vi "Main.vi"() -> ()   [LabVIEW 2010]
uses:
  typedefs/state_cluster.ctl
  typedefs/state_enum.ctl
  <vilib>/DAQmx/write.llb/DAQmx Write (Analog 1D DBL NChan 1Samp).vi
  <vilib>/DAQmx/create/channels.llb/DAQmx Create Channel (AO-Voltage-Basic).vi
  <vilib>/DAQmx/configure/timing.llb/DAQmx Timing (Sample Clock).vi
  <vilib>/DAQmx/miscellaneous.llb/DAQmx Fill In Error Info.vi
panel:
  in  "Zeit pro Zelle":dbl
  out "Internal quit":bool
  out "Pfadlänge":dbl
  out "Image":picture
  in  "Quit":bool
  out "Signal Qualität":dbl(slide) scale=0.0..10.0
  out "Anzahl Neurone":u16(slide) scale=0.0..200.0
  out "Scan Geschwindigkeit":dbl(slide) scale=0.0..1.0
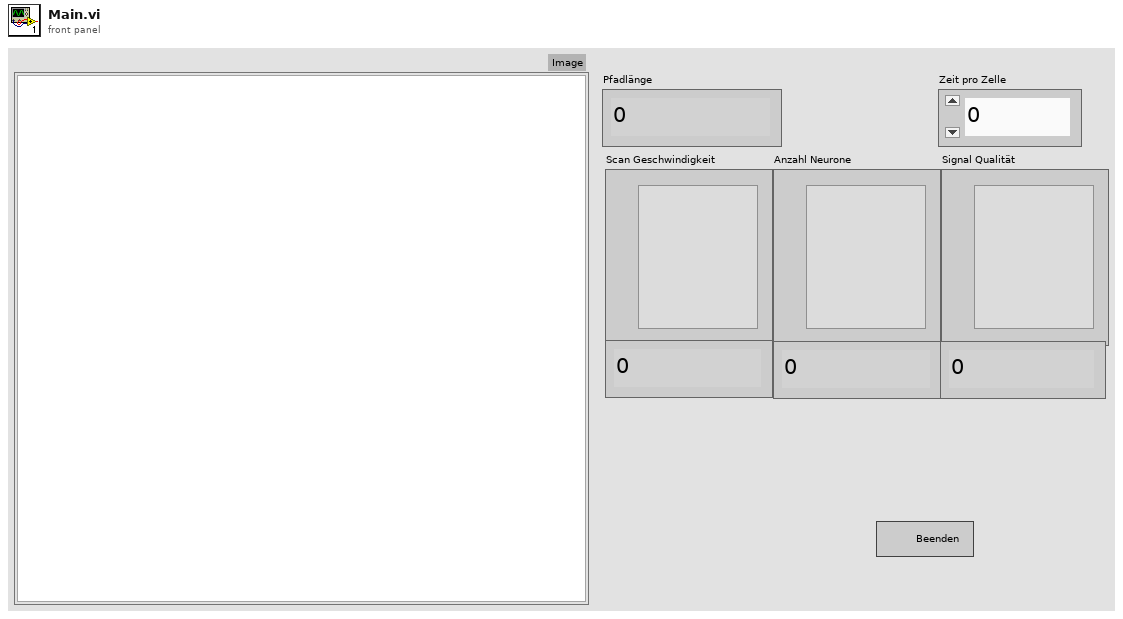
[diagram p1: front panel]
types:
  T1 = typedef "state_cluster.ctl" = cluster{"State":T2, "variant":variant}
  T2 = typedef "state_enum.ctl" = enum16{"Init", "StartSetting", "Moving", "SetNeuron", "FinishSetting", "Quit"}
  T3 = cluster{"Width":u16, "Style":enum32{"Solid", "Dash", "Dot", "DashDot", "DashDotDot"}}
  T4 = typedef "LVBoundsTypeDef.ctl" = cluster{"Width":u32, "Height":u32}
  T5 = typedef "LVMouseTypeDef.ctl" = cluster{"Mouse Position":cluster{"X":i32, "Y":i32}, "Mouse Modifiers":cluster{"Button Down":bool, "Shift Mod":bool, "Menu Mod":bool, "Option Mod":bool}}
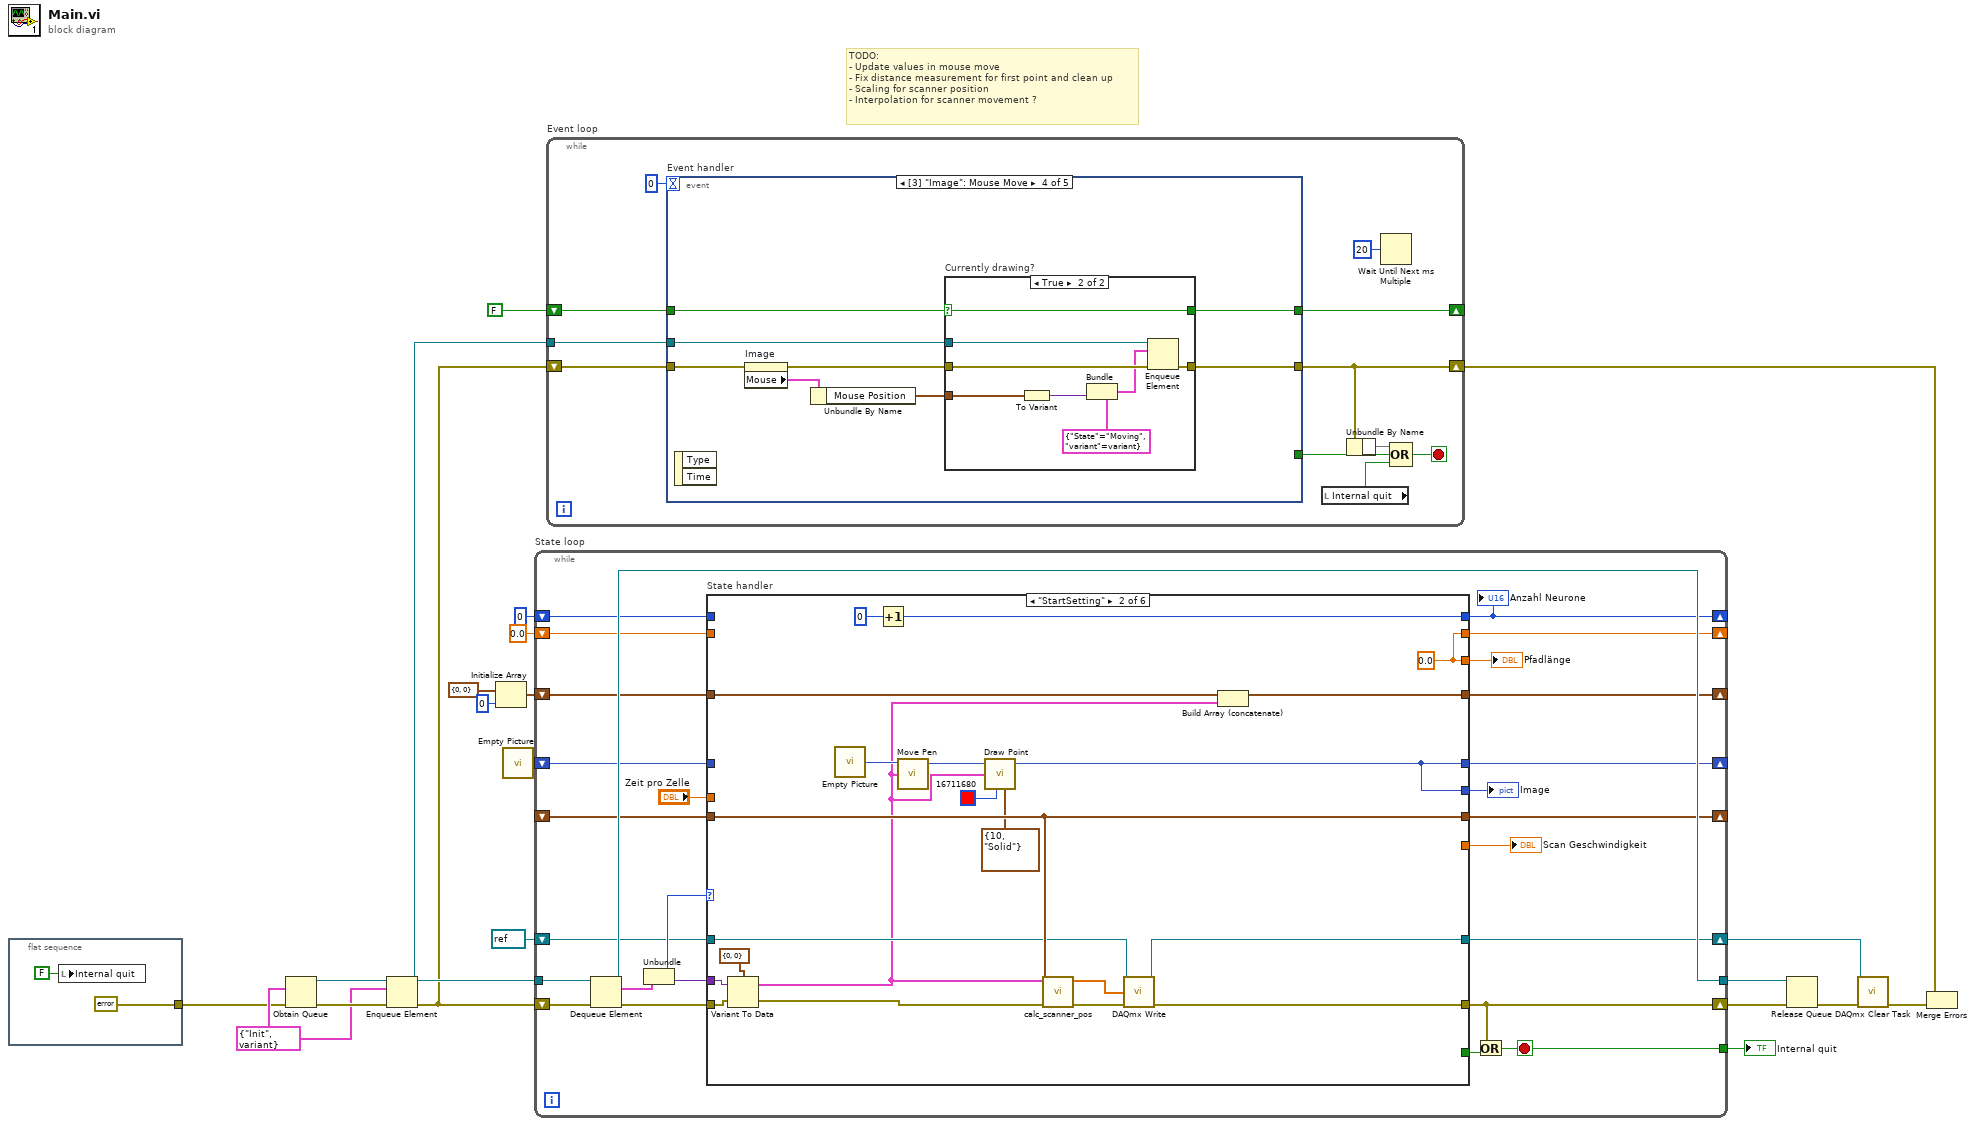
[diagram p0: block diagram]
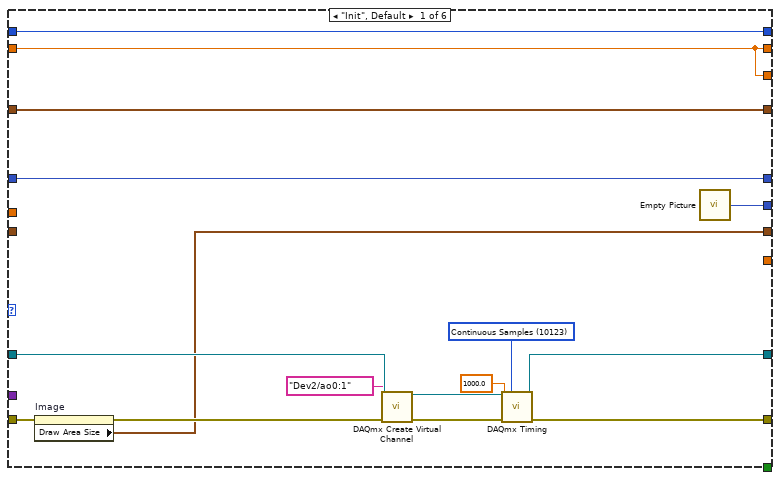
[diagram p2: hidden frame]
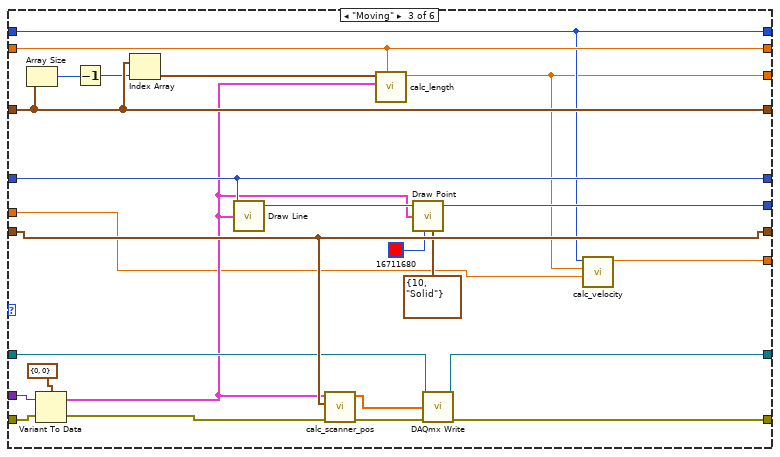
[diagram p3: hidden frame]
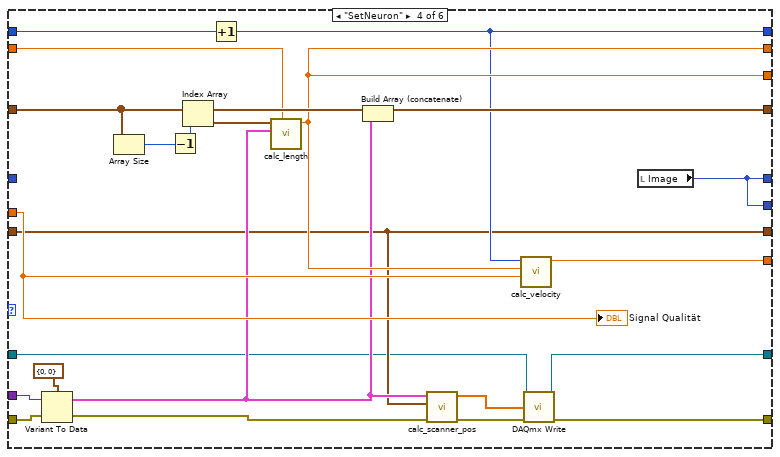
[diagram p4: hidden frame]
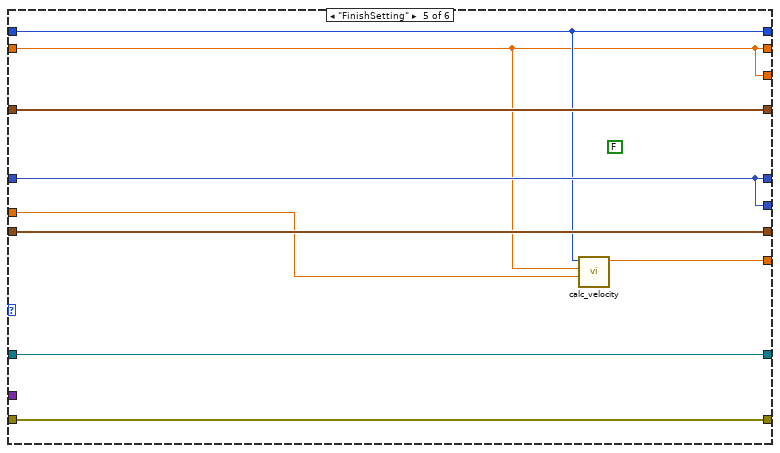
[diagram p5: hidden frame]
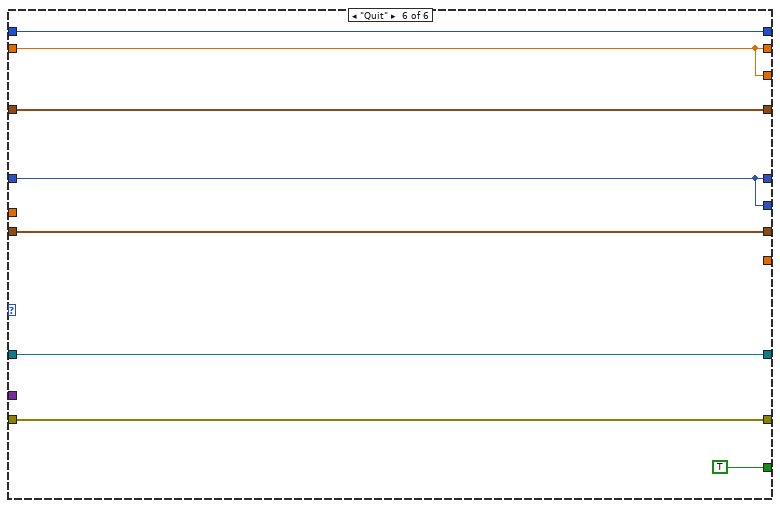
[diagram p6: hidden frame]
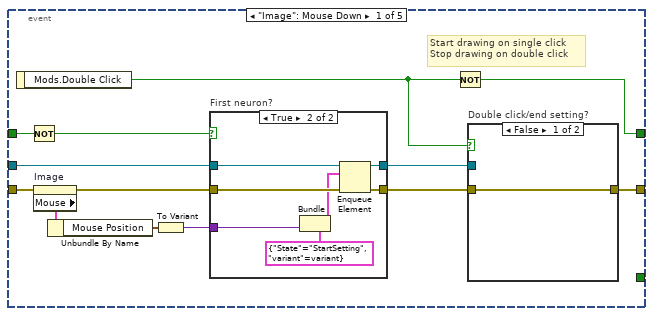
[diagram p7: hidden frame]
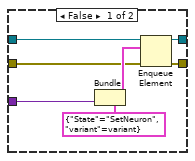
[diagram p8: hidden frame]
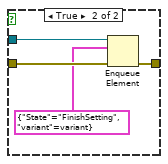
[diagram p9: hidden frame]
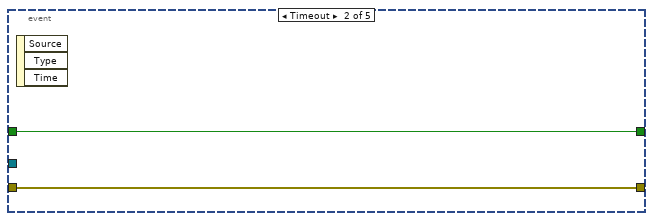
[diagram p10: hidden frame]
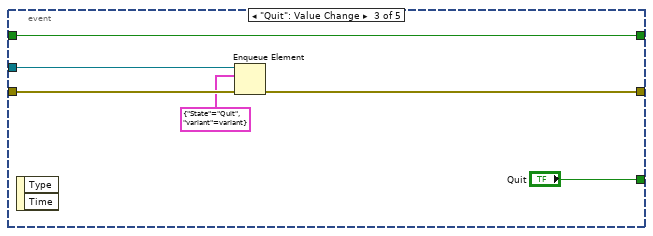
[diagram p11: hidden frame]
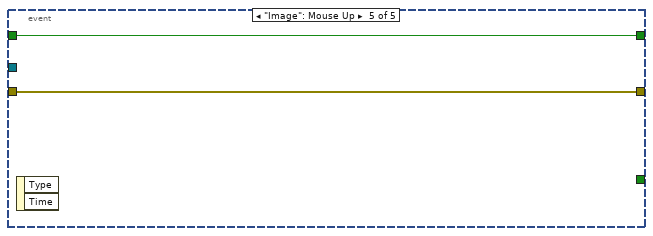
[diagram p13: hidden frame]
diagram:
  w18 = T1 {"State"=enum."Init", "variant"=variant}
  # "TODO:\n- Update values in mouse move\n- Fix distance measurement for first point and clean up\n- Scaling for scanner position\n- Interpolation for scanner movement ?"
  n1 = flat-sequence {
    tunnel: [errorcluster {"status"=FALSE, "code"=0, "source"=""} ("error in (no error)")] -> w5
    frame #0 {
      n2 = local write "Internal quit"(FALSE ("Internal quit")) -> ()
    }
  }
  n3 = Obtain Queue(element data type=w18, error in (no error)=w5) -> (queue out=w19:refnum<queue>, error out=w20:errorcluster)  [unwired: 3 in, 1 out]
  n4 = Enqueue Element(queue=w19, element=w18, error in (no error)=w20) -> (queue out=w10:refnum<queue>, error out=w8:errorcluster)  [unwired: 1 in, 1 out]
  n5 = Initialize Array(cluster{"X":i32, "Y":i32} {"X"=0, "Y"=0} ("Mouse Position"), 0 ("dimension size")) -> (w11:cluster{"X":i32, "Y":i32}[])
  n6 = call "Empty Picture"() -> ("empty picture"=w9:picture)
  n7 = while "State loop" {
    shift-right: [w42] -> w17
    shift-left: w8 -> [w49]
    tunnel: w10 -> [w47]
    tunnel: [w43] -> w16
    shift-right: [w30] -> _
    shift-left: u16 0 -> [w40]
    shift-right: [w34] -> _
    shift-left: 0.0 -> [w39]
    shift-right: [w37] -> _
    shift-left: w11 -> [w38]
    shift-right: [w35] -> _
    shift-left: w9 -> [w36]
    tunnel: [w31] -> w7
    shift-right: [w28] -> w1
    shift-left: refnum<k21> refnum ("task out") -> [w27]
    shift-right: [w26] -> _
    shift-left: _ -> [w25]
    stop <- w31 stop-if-true
    n8 = Dequeue Element(queue=w47, error in (no error)=w49) -> (queue out=w43:refnum<queue>, element=w46:T1, error out=w48:errorcluster)  [unwired: 1 in, 1 out]
    n9 = Unbundle(w46) -> ("State"=w45:T2, "variant"=w44:variant)
    n10 = case "State handler" shown="\"StartSetting\"" w45 {
      tunnel: w48 -> [w57 w85 w110 w133 w143 w145]
      tunnel: [w60 w77 w100 w118 w143 w145] -> w42
      tunnel: w44 -> [_ w84 w109 w132 _ _]
      tunnel: [_ _ _ _ _ TRUE] -> w41
      tunnel: w40 -> [w65 _ w89 w134 w137 w150]
      tunnel: [w65 w81 w89 w122 w137 w150] -> w30
      tunnel: w39 -> [w62 _ w107 w128 w136 w148]
      tunnel: w38 -> [w64 w72 w106 w129 w142 w149]
      tunnel: [w64 w73 w106 w130 w142 w149] -> w37
      tunnel: [w62 w82 w107 w123 w136 w148] -> w34
      tunnel: w36 -> [w63 _ w108 _ w141 w147]
      tunnel: [w63 w70 w108 w127 w141 w147] -> w35
      tunnel: [w61 w70 w94 w127 w141 w147] -> w33
      tunnel: [w62 w82 w88 w123 w136 w148] -> w32
      tunnel: "Zeit pro Zelle" -> [_ _ w87 w121 w135 _]
      tunnel: [w59 w75 w97 w114 w140 w146] -> w28
      tunnel: w27 -> [w58 w76 w98 w115 w140 w146]
      tunnel: [w55 w79 w99 w116 w139 w144] -> w26
      tunnel: w25 -> [_ w79 w99 w116 w139 w144]
      tunnel: [_ _ w90 w112 w138 _] -> w24
      frame "Init", Default {
        w53 = 10123 items=["Finite Samples"=10178, "Continuous Samples"=10123, "Hardware Timed Single Point"=12522] ("sample mode")
        n11 = property on="Image" class="Pict"(error in=w57) -> (error out=w56:errorcluster, "Draw Area Size"=w55:T4)  [unwired: 1 in, 1 out]
        n12 = call-poly <vilib>:"DAQmx Create Virtual Channel.vi"("task in"=w58, "physical channels"=tag "Dev2/ao0:1", "error in"=w56) -> ("task out"=w52:refnum<k21>, "error out"=w54:errorcluster)  [unwired: 11 in]
        n13 = call-poly <vilib>:"DAQmx Timing.vi"("task/channels in"=w52, "sample mode"=w53, "rate"=1000.0, "error in"=w54) -> ("task out"=w59:refnum<k21>, "error out"=w60:errorcluster)  [unwired: 10 in]
        n14 = call "Empty Picture"() -> ("empty picture"=w61:picture)
      }
      frame "StartSetting" {
        w82 = 0.0
        n15 = Variant To Data(error in=w85, Variant=w84, type=cluster{"X":i32, "Y":i32} {"X"=0, "Y"=0} ("Mouse Position")) -> (error out=w80:errorcluster, data=w69:cluster{})
        n16 = call "Empty Picture"() -> ("empty picture"=w83:picture)
        n17 = Increment(x=u16 0) -> (x+1=w81:u16)
        n18 = call <vilib>:"Move Pen.vi"("new position"=w69, "picture"=w83) -> ("new picture"=w71:picture)  [unwired: 3 in]
        n19 = call <vilib>:"Draw Point.vi"("picture"=w71, "point(x,y)"=w69, "color(black)"=u32 16711680, "pen"=T3 {"Width"=10, "Style"=enum."Solid"}) -> ("new picture"=w70:picture)  [unwired: 5 in]
        n20 = call "calc_scanner_pos.vi"("error in (no error)"=w80, "Draw Area Size"=w79, "Mouse position"=w69) -> ("error out"=w78:errorcluster, "Scanner position"=w74:dbl[])  [unwired: 7 in]
        n21 = call-poly <vilib>:"DAQmx Write.vi"("task/channels in"=w76, "data"=w74, "error in"=w78) -> ("task out"=w75:refnum<k21>, "error out"=w77:errorcluster)  [unwired: 10 in, 1 out]
        n22 = Build Array (concatenate)(w72, w69) -> (w73:cluster{"X":i32, "Y":i32}[])
      }
      frame "Moving" {
        n23 = Array Size(array=w106) -> (size(s)=w105:i32)
        n24 = Variant To Data(error in=w110, Variant=w109, type=cluster{"X":i32, "Y":i32} {"X"=0, "Y"=0} ("Mouse Position")) -> (error out=w101:errorcluster, data=w93:cluster{})
        n25 = Decrement(x=w105) -> (x-1=w104:i32)
        n26 = Index Array(array=w106, index=w104) -> (element=w103:cluster{"X":i32, "Y":i32})
        n27 = call <vilib>:"Draw Line.vi"("picture"=w108, "end point"=w93) -> ("new picture"=w95:picture)  [unwired: 7 in]
        n28 = call "calc_scanner_pos.vi"("error in (no error)"=w101, "Draw Area Size"=w99, "Mouse position"=w93) -> ("error out"=w102:errorcluster, "Scanner position"=w96:dbl[])  [unwired: 7 in]
        n29 = call "calc_length.vi"("Old length"=w107, "Current point"=w93, "Last point"=w103) -> ("New length"=w88:dbl)  [unwired: 8 in]
        n30 = call <vilib>:"Draw Point.vi"("picture"=w95, "point(x,y)"=w93, "color(black)"=u32 16711680, "pen"=T3 {"Width"=10, "Style"=enum."Solid"}) -> ("new picture"=w94:picture)  [unwired: 5 in]
        n31 = call-poly <vilib>:"DAQmx Write.vi"("task/channels in"=w98, "data"=w96, "error in"=w102) -> ("task out"=w97:refnum<k21>, "error out"=w100:errorcluster)  [unwired: 10 in, 1 out]
        n32 = call "calc_velocity.vi"("Time per cell"=w87, "Path length"=w88, "Neurons"=w89) -> ("Velocity"=w90:dbl)  [unwired: 8 in]
      }
      frame "SetNeuron" {
        n33 = Variant To Data(error in=w133, Variant=w132, type=cluster{"X":i32, "Y":i32} {"X"=0, "Y"=0} ("Mouse Position")) -> (error out=w119:errorcluster, data=w117:cluster{})
        n34 = Array Size(array=w129) -> (size(s)=w125:i32)
        n35 = Decrement(x=w125) -> (x-1=w126:i32)
        n36 = Index Array(array=w129, index=w126) -> (element=w124:cluster{"X":i32, "Y":i32})
        n37 = Increment(x=w134) -> (x+1=w122:u16)
        n38 = call "calc_length.vi"("Old length"=w128, "Current point"=w117, "Last point"=w124) -> ("New length"=w123:dbl)  [unwired: 8 in]
        n39 = Build Array (concatenate)(w129, w117) -> (w130:cluster{"X":i32, "Y":i32}[])
        n40 = call "calc_scanner_pos.vi"("error in (no error)"=w119, "Draw Area Size"=w116, "Mouse position"=w117) -> ("error out"=w120:errorcluster, "Scanner position"=w113:dbl[])  [unwired: 7 in]
        n41 = call "calc_velocity.vi"("Time per cell"=w121, "Path length"=w123, "Neurons"=w122) -> ("Velocity"=w112:dbl)  [unwired: 8 in]
        n42 = call-poly <vilib>:"DAQmx Write.vi"("task/channels in"=w115, "data"=w113, "error in"=w120) -> ("task out"=w114:refnum<k21>, "error out"=w118:errorcluster)  [unwired: 10 in, 1 out]
        n43 = local read "Image"() -> (w127:picture)
        "Signal Qualität" <- w121
      }
      frame "FinishSetting" {
        (unwired) FALSE
        n44 = call "calc_velocity.vi"("Time per cell"=w135, "Path length"=w136, "Neurons"=w137) -> ("Velocity"=w138:dbl)  [unwired: 8 in]
      }
      frame "Quit" {
      }
    }
    "Image" <- w33
    "Pfadlänge" <- w32
    "Anzahl Neurone" <- w30
    "Scan Geschwindigkeit" <- w24
    n45 = Or(x=w42, y=w41) -> (x .or. y?=w31:bool)
  }
  "Internal quit" <- w7
  n46 = while "Event loop" {
    shift-right: [w158] -> w6
    shift-left: w8 -> [w162]
    shift-right: [w161] -> _
    shift-left: FALSE -> [w160]
    tunnel: w10 -> [w156]
    stop <- w157 stop-if-true
    n47 = event "Event handler" shown="[3] \"Image\": Mouse Move" {
      selector: _ -> [_ _ _ _ _]
      dyn-events: _ -> [_ _ _ _ _]
      timeout: 0 -> [_ _ _ _ _]
      tunnel: w162 -> [w175 w196 w200 w209 w222]
      tunnel: [w170 w196 w199 w210 w222] -> w158
      tunnel: [w173 w195 w201 w203 w221] -> w161
      tunnel: w160 -> [w166 w195 w201 w207 w221]
      tunnel: [_ _ "Quit" _ _] -> w159
      tunnel: w156 -> [w168 _ w198 w204 _]
      event "Image": Mouse Down {
        # "Start drawing on single click\nStop drawing on double click"
        n48 = event-data() -> ("Mods.Double Click"=w171:bool)  [unwired: 1 in]
        n49 = Not(x=w166) -> (.not. x?=w167:bool)
        n50 = property on="Image" class="Pict"(error in=w175) -> (error out=w169:errorcluster, "Mouse"=w174:T5)  [unwired: 1 in, 1 out]
        n51 = Unbundle By Name(w174) -> ("Mouse Position"=w172:cluster{"X":i32, "Y":i32})
        n52 = To Variant(anything=w172) -> (Variant=w165:variant)
        n53 = case "First neuron?" shown="True" w167 {
          tunnel: w169 -> [w180 w189]
          tunnel: [w179 w188] -> w164
          tunnel: w168 -> [w178 w187]
          tunnel: [w177 w186] -> w163
          tunnel: w165 -> [w176 w184]
          frame False {
            n54 = Bundle(cluster=T1 {"State"=enum."SetNeuron", "variant"=variant} ("element"), "variant"=w176) -> (w181:T1)  [unwired: 1 in]
            n55 = Enqueue Element(queue=w178, element=w181, error in (no error)=w180) -> (queue out=w177:refnum<queue>, error out=w179:errorcluster)  [unwired: 1 in, 1 out]
          }
          frame True {
            n56 = Bundle(cluster=T1 {"State"=enum."StartSetting", "variant"=variant} ("element"), "variant"=w184) -> (w183:T1)  [unwired: 1 in]
            n57 = Enqueue Element(queue=w187, element=w183, error in (no error)=w189) -> (queue out=w186:refnum<queue>, error out=w188:errorcluster)  [unwired: 1 in, 1 out]
          }
        }
        n58 = Not(x=w171) -> (.not. x?=w173:bool)
        n59 = case "Double click/end setting?" shown="False" w171 {
          tunnel: w164 -> [w190 w194]
          tunnel: [w190 w193] -> w170
          tunnel: w163 -> [_ w192]
          frame False {
          }
          frame True {
            n60 = Enqueue Element(queue=w192, element=T1 {"State"=enum."FinishSetting", "variant"=variant}, error in (no error)=w194) -> (error out=w193:errorcluster)  [unwired: 1 in, 2 out]
          }
        }
      }
      event Timeout {
        n61 = event-data() -> ()  [unwired: 1 in, 3 out]
      }
      event "Quit": Value Change {
        n62 = event-data() -> ()  [unwired: 1 in, 2 out]
        n63 = Enqueue Element(queue=w198, element=T1 {"State"=enum."Quit", "variant"=variant}, error in (no error)=w200) -> (error out=w199:errorcluster)  [unwired: 1 in, 2 out]
      }
      event "Image": Mouse Move {
        n64 = event-data() -> ()  [unwired: 1 in, 2 out]
        n65 = property on="Image" class="Pict"(error in=w209) -> (error out=w208:errorcluster, "Mouse"=w206:T5)  [unwired: 1 in, 1 out]
        n66 = Unbundle By Name(w206) -> ("Mouse Position"=w205:cluster{"X":i32, "Y":i32})
        n67 = case "Currently drawing?" shown="True" w207 {
          selector: w207 -> [w211 w213]
          tunnel: [w212 w219] -> w210
          tunnel: w208 -> [w212 w220]
          tunnel: w205 -> [_ w215]
          tunnel: w204 -> [_ w218]
          tunnel: [w211 w213] -> w203
          frame False {
          }
          frame True {
            n68 = To Variant(anything=w215) -> (Variant=w216:variant)
            n69 = Bundle(cluster=T1 {"State"=enum."Moving", "variant"=variant} ("element"), "variant"=w216) -> (w214:T1)  [unwired: 1 in]
            n70 = Enqueue Element(queue=w218, element=w214, error in (no error)=w220) -> (error out=w219:errorcluster)  [unwired: 1 in, 2 out]
          }
        }
      }
      event "Image": Mouse Up {
        n71 = event-data() -> ()  [unwired: 1 in, 2 out]
      }
    }
    n72 = local read "Internal quit"() -> (w155:bool)
    n73 = Wait Until Next ms Multiple(millisecond multiple=u32 20) -> ()  [unwired: 1 out]
    n74 = Compound Arithmetic op=OR(w152, w159, w155) -> (w157:bool)
  }
  n75 = Unbundle By Name(w158) -> (w152)
  n76 = Release Queue(queue=w16, error in (no error)=w17) -> (error out=w3:errorcluster)  [unwired: 1 in, 2 out]
  n77 = call <vilib>:"DAQmx Clear Task.vi"("task in"=w1, "error in"=w3) -> ("error out"=w2:errorcluster)  [unwired: 13 in]
  n78 = Merge Errors(w6, w2) -> ()  [unwired: 1 out]
